vi "Read Variant.vi"(8 "error in (no error)":errorcluster, 9 "element data type":variant, 10 "Tag Name":string, 11 "Current Value Table in":refnum<class "Current Value Table.lvclass">) -> (0 "error out":errorcluster, 2 "value":variant, 3 "Current Value Table out":refnum<class "Current Value Table.lvclass">)   [LabVIEW 2024, in "Current Value Table.lvlib" / "Current Value Table.lvclass"]
uses:
  Current Value Table.lvclass
  iCVT_Item/iCVT_Item.lvclass
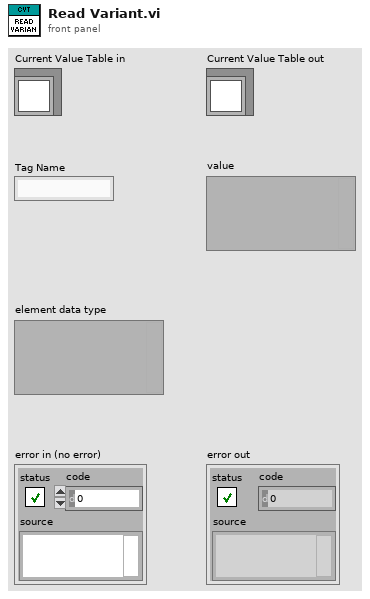
[diagram p1: front panel]
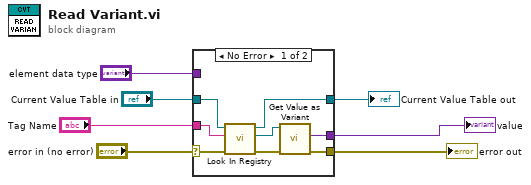
[diagram p0: block diagram]
diagram:
  n1 = case shown="No Error" "error in (no error)" {
    selector: "error in (no error)" -> [w10 w17]
    tunnel: [w11 w17] -> w6
    tunnel: [w8 w16] -> w4
    tunnel: "Current Value Table in" -> [w15 w16]
    tunnel: "Tag Name" -> [w14 _]
    tunnel: [w12 _] -> w2
    tunnel: "element data type" -> [_ _]
    frame No Error {
      n2 = call-dynamic "Look In Registry.vi"("error in (no error)"=w10, "Tag Name"=w14, "Current Value Table in"=w15) -> ("error out"=w9:errorcluster, "CVT_Item out"=w13:refnum<class "iCVT_Item.lvclass">, "Current Value Table out"=w8:refnum<class "Current Value Table.lvclass">)  [unwired: 5 in, 1 out]
      n3 = call-dynamic "Get Value as Variant.vi"("error in (no error)"=w9, "iCVT_Item in"=w13) -> ("error out"=w11:errorcluster, "data"=w12:variant)  [unwired: 7 in, 1 out]
    }
    frame Error {
    }
  }
  "error out" <- w6
  "Current Value Table out" <- w4
  "value" <- w2
